vi "Write Count.vi"(8 "error in (no error)":errorcluster, 10 "Data Count":u32, 11 "Tracker Data in":refnum<class "Tracker Data.lvclass">) -> (0 "error out":errorcluster, 3 "Tracker Data out":refnum<class "Tracker Data.lvclass">)   [LabVIEW 2020, in "Data Tracker.lvlib" / "Tracker Data.lvclass"]
doc: "Write Data Count to the class."
uses:
  Tracker Data.lvclass
  Tracker Data.lvclass/Tracker Data.ctl
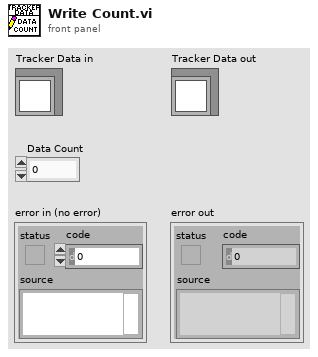
[diagram p1: front panel]
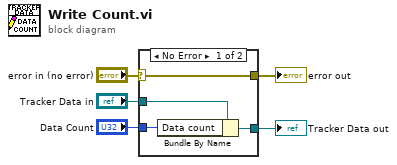
[diagram p0: block diagram]
diagram:
  n1 = case shown="No Error" "error in (no error)" {
    selector: "error in (no error)" -> [w9 w10]
    tunnel: [w9 w10] -> w4
    tunnel: [w7 w11] -> w2
    tunnel: "Tracker Data in" -> [w8 w11]
    tunnel: "Data Count" -> [w6 _]
    frame No Error {
      n2 = Bundle By Name(cluster=w8, "Data count"=w6) -> (w7:refnum<class "Tracker Data.lvclass">)
    }
    frame Error {
    }
  }
  "error out" <- w4
  "Tracker Data out" <- w2
